vi "Rotate 2D stats.vi"(6 "uv":dbl, 7 "Rotation angle (deg)":dbl, 8 "v^2":dbl, 9 "u^2":dbl, 10 "V":dbl, 11 "U":dbl) -> (0 "v~^2":dbl, 1 "u~^2":dbl, 2 "V~":dbl, 3 "U~":dbl, 4 "u~v~":dbl)   [LabVIEW 2014]
panel:
  # "Anti-clockwise looking into axis of rotation. Rotation is about the axis perpendicular to the plane of the measured velocity vector."
  # "These stats may be weighted or un-weighted. The only constraint is that the rotation angle is constant over all samples."
  # "PN 21/10/2014"
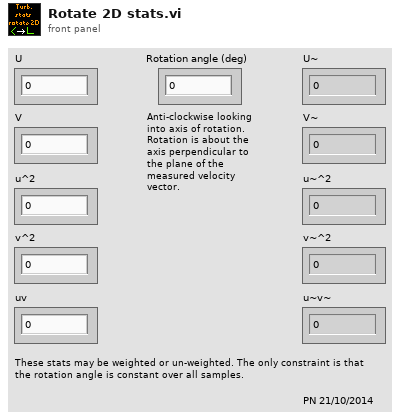
[diagram p1: front panel]
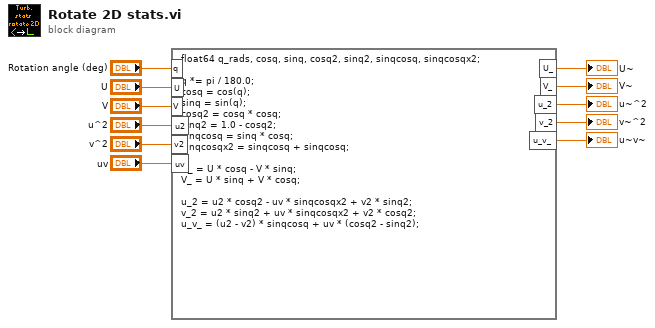
[diagram p0: block diagram]
diagram:
  n1 = formula code="float64 q_rads, cosq, sinq, cosq2, sinq2, sinqcosq, sinqcosqx2;\n\nq *= pi / 180.0;\ncosq = cos(q);\nsinq = sin(q);\ncosq2 = cosq * cosq;\nsinq2 = 1.0 - cosq2;\nsinqcosq = sinq * cosq;\nsinqcosqx2 = sinqcosq + sinqcosq;\n\nU_ = U * cosq - V * sinq;\nV_ = U * sinq + V * cosq;\n\nu_2 = u2 * cosq2 - uv * sinqcosqx2 + v2 * sinq2;\nv_2 = u2 * sinq2 + uv * sinqcosqx2 + v2 * cosq2;\nu_v_ = (u2 - v2) * sinqcosq + uv * (cosq2 - sinq2);"("U"="U", "V"="V", "u2"="u^2", "v2"="v^2", "uv"="uv", "q"="Rotation angle (deg)") -> ("U_"=→"U~":dbl, "V_"=→"V~":dbl, "u_2"=→"u~^2":dbl, "v_2"=→"v~^2":dbl, "u_v_"=→"u~v~":dbl)
